vi "HOST_425.vi"() -> ()   [LabVIEW 2018]
uses:
  <vilib>/userdefined/High Color/nirio_resource_hc.ctl
  <instrlib>/niDCPower/nidcpower.llb/niDCPower Measurement Type.ctl
  <vilib>/FPGAPlugInAG/PXI-7953R/niLvFpga_Open_PXI-7953R.vi
  <vilib>/rvi/interface/common/dynamic/niFpgaDynamicAddResources.vi
  <vilib>/FPGAPlugInAG/Dynamic/niLvFpga_Reset_Dynamic.vi
  <vilib>/FPGAPlugInAG/Dynamic/niLvFpga_Run_Dynamic.vi
  <vilib>/Utility/error.llb/Error Cluster From Error Code.vi
  <vilib>/rvi/errors/niLvFpgaAdjustHostInterfaceError.vi
  <vilib>/FPGAPlugInAG/Dynamic/niLvFpga_Close_Dynamic.vi
  <vilib>/rvi/interface/nirviOpenFPGA/nirviOpenFPGA.xnode
  FPGA Bitfiles/IMX425LLJ_FPGATarget_Target0505_scNoFcOBk0w.lvbitx
  <vilib>/rvi/interface/nirviMethod/nirviMethod.xnode
  <vilib>/rvi/interface/nirviReadWriteControl/nirviReadWriteControl.xnode
  <vilib>/rvi/interface/nirviCloseFPGA/nirviCloseFPGA.xnode
  <vilib>/rvi/interface/Simulation/niFpgaSimulationCallBeginRW.vi
  <vilib>/FPGAPlugInAG/Dynamic/niLvFpga_ReadFifo_Dynamic.vi
  <vilib>/rvi/errors/niLvFpgaMergeErrorWithErrorCode.vi
  NiFpgaLv.dll
  <vilib>/FPGAPlugInAG/Dynamic/niLvFpga_StartFifo_Dynamic.vi
  <vilib>/FPGAPlugInAG/Dynamic/niLvFpga_WriteFifo_Dynamic.vi
panel:
  in  "Регистры":u32[](array[numeric])=[4194304, 4206720, 4205568, 4209664, 4197129, 4229936, 4213512, 4246304, 4205320, 4238224, 4221696, 4201291, 4233984, 4209536, 4212500, 4245304, 12582912, 12591104, 12623872, 12583936, 12616704, 12600320, 12633088, 12592128, 12624896, 12608512, 12641280, 12588032, 12620800, 12604416, 12637184, 12596224, 12628992, 12612608, 12645376, 12585984, 12618752, 12602368, 12635136, 12594176, 12626944, 12610560, 12643328, 12590080, 12622848, 12606464, 12639232, 12598272, 12631040, 12614656, 12647424, 12583424, 12616192, 12599808, 12632576, 12591616, 12624384, 12608000, 12640768, 12587520, 12620288, 12603904, 12636672, 12595712, 12628480, 12612096, 12644864, 12585472, 12618240, 12601856, 12634624, 12593664, 12626432, 12610048, 12642816, 12589568, 12622336, 12605952, 12638720, 12597760, 12630528, 12614144, 12646912, 2097188, 2105344, 2098186, 2130948, 2106378, 2139140, 2122949, 2100248, 2133016, 2116800, 2097716, 2130432, 2114048, 6291584, 6294656, 6335488, 6315008, 6306819, 6300352, 6332960, 6299136, 6331904, 6315520, 6348288, 6307328, 6340096, 6323712, 6291712, 6324480, 6308096, 6340864, 6299904, 6332672, 6316288, 14696448, 14682112, 14690304, 14723072, 14680892, 14713600, 14693320, 14725888, 14709688, 14742272, 1064960, 1097728, 1069064, 1101824, 1077288, 1110016, 1067248, 1099776, 1075296, 1107968, 1071152, 1103872, 1070080, 1102848, 1078288, 1111040, 1076264, 1108992, 1080362, 1113088, 1065520, 1098240, 1067520, 1100288, 1075728, 1108480, 1071624, 1104384, 1079848, 1112576, 1074784, 1107456, 13639680, 13632512, 13665344, 13648976, 13640959, 13673726, 13657088, 13636616, 13653000, 13644808, 13634645, 13667328, 13650950, 13683712, 13642752, 13675520, 13659136, 13691904, 13638656, 13671424, 13655040, 13687808, 13632192, 13664768, 15209792, 15242496]
  out "LED_char":dbl(graph)=-9.950040532110056e-06
  out "Память":i32
  out "Image":T1(plugin-control)
  in  "Хватит ждать!":bool
  out "Выкачали из памяти":bool
  out "SEU":u32
  in  "Upd_WR":bool
  out "FIFO_READ":u32
  in  "W(T)/R(F)":bool
  in  "Адрес":u8
  in  "Кол-во":u16=185
  out "НИ":bool
  out "READ":u8[](array[numeric])
  out "Прошили":bool
  in  "SPI":bool
  in  "Обнулить сбои":bool
  in  "Проверка сбоев":bool
  out "世男":bool
  in  "Период опроса, мс":u32=1
  in  "OVDD, V":dbl=1.8 caption="voltage level" format="%_6p"
  in  "OVDD_curlim":dbl=0.1 caption="current limit" format="%_6p"
  out "OVDD_char":dbl(graph)=1.5967060684808935e-06
  in  "3,3_LVDS, V":dbl=3.3 caption="voltage level" format="%_6p"
  in  "AVDD, V":dbl=3.3 caption="voltage level" format="%_6p"
  in  "DVDD, V":dbl=1.2 caption="voltage level" format="%_6p"
  in  "3,3_LVDS_curlim":dbl=0.2 caption="current limit" format="%_6p"
  in  "AVDD_curlim":dbl=1.0 caption="current limit" format="%_6p"
  in  "DVDD_curlim":dbl=1.0 caption="current limit" format="%_6p"
  in  "LED_curlim":dbl=0.1 caption="current limit" format="%_6p"
  in  "LED, V":dbl=-1.3 caption="voltage level" format="%_6p"
  out "3,3_LVDS_char":dbl(graph)=-0.007753012065680951
  out "AVDD_char":dbl(graph)=9.424895165128459e-05
  out "DVDD_char":dbl(graph)=-9.950040532110056e-06
  out "DVDD_cur":dbl caption="measurement" format="%_6g"
  out "LED_cur":dbl caption="measurement" format="%_6g"
  in  "SEL_Time, ms":u32=100
  in  "OVDD_selcur":dbl=0.01 caption="current limit" format="%_6p"
  in  "AVDD_selcur":dbl=0.6 caption="current limit" format="%_6p"
  in  "DVDD_selcur":dbl=0.9 caption="current limit" format="%_6p"
  out "AVDD_cur":dbl caption="measurement" format="%_6g"
  out "3,3_LVDS_cur":dbl caption="measurement" format="%_6g"
  out "OVDD_cur":dbl caption="measurement" format="%_6g"
  in  "MOVIE":bool
  in  "FRAME!":bool
  out "SEL":bool
  in  "SIM_SEL":bool
  out "OVDD":u16
  out "AVDD":u16
  out "DVDD":u16
  out "OVDD":bool
  out "AVDD":bool
  out "DVDD":bool
  in  "Стоп":bool
  in  "Питание":bool
  in  "LED":bool caption="output enabled"
  in  "0":refnum<k15>="PXI1Slot2" caption="1"
  in  "1":refnum<k15>="PXI1Slot3"
  in  "resource name 2":T2="PXI1Slot6"
  in  "SEU":path=path "C:/LabView_PRJ/GMAX0505/SEU"
  in  "SEL":path=path "C:/LabView_PRJ/GMAX0505/SEL"
  out "Номер образца":string="1"
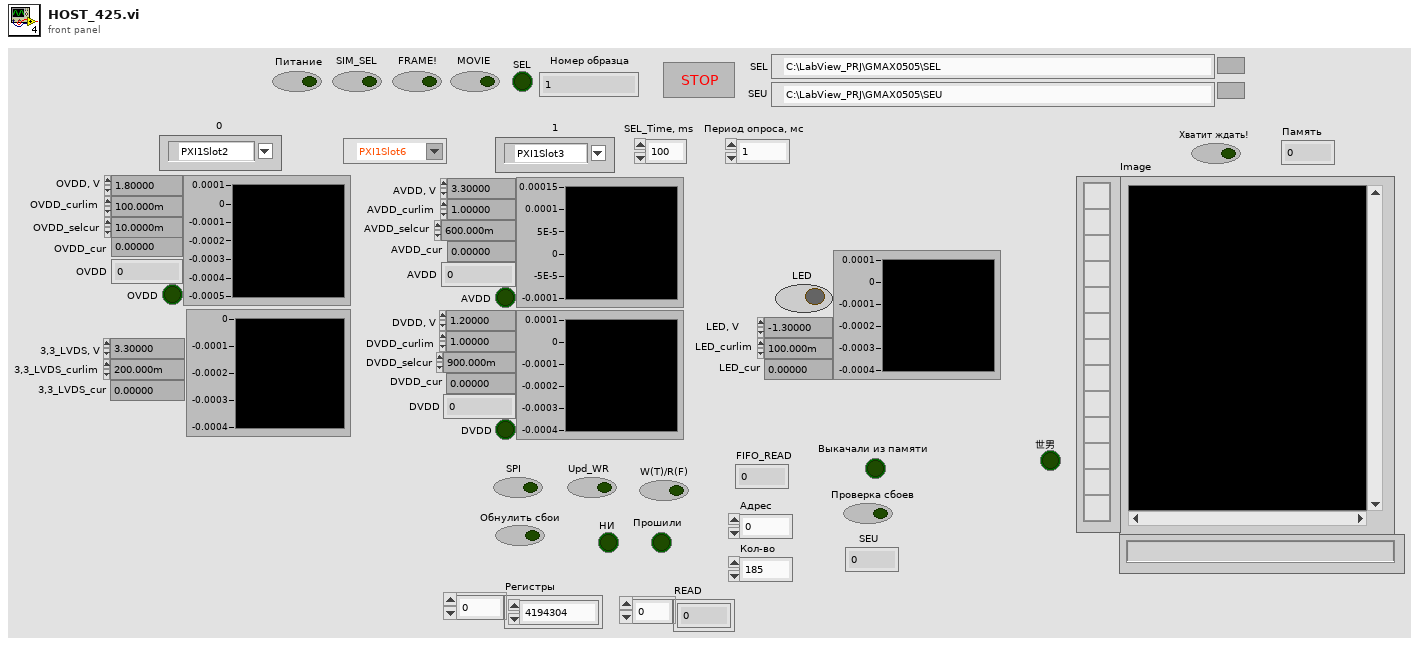
[diagram p1: front panel]
types:
  T1 = typedef "IMAQ Image.ctl" = refnum<image>
  T2 = typedef "nirio_resource_hc.ctl" = tag
  T3 = enum16{"open", "replace", "create", "open or create", "replace or create", "replace or create with confirmation"}
  T4 = typedef "Image Type" = u32
  T5 = typedef "niDCPower Measurement Type.ctl" = i32
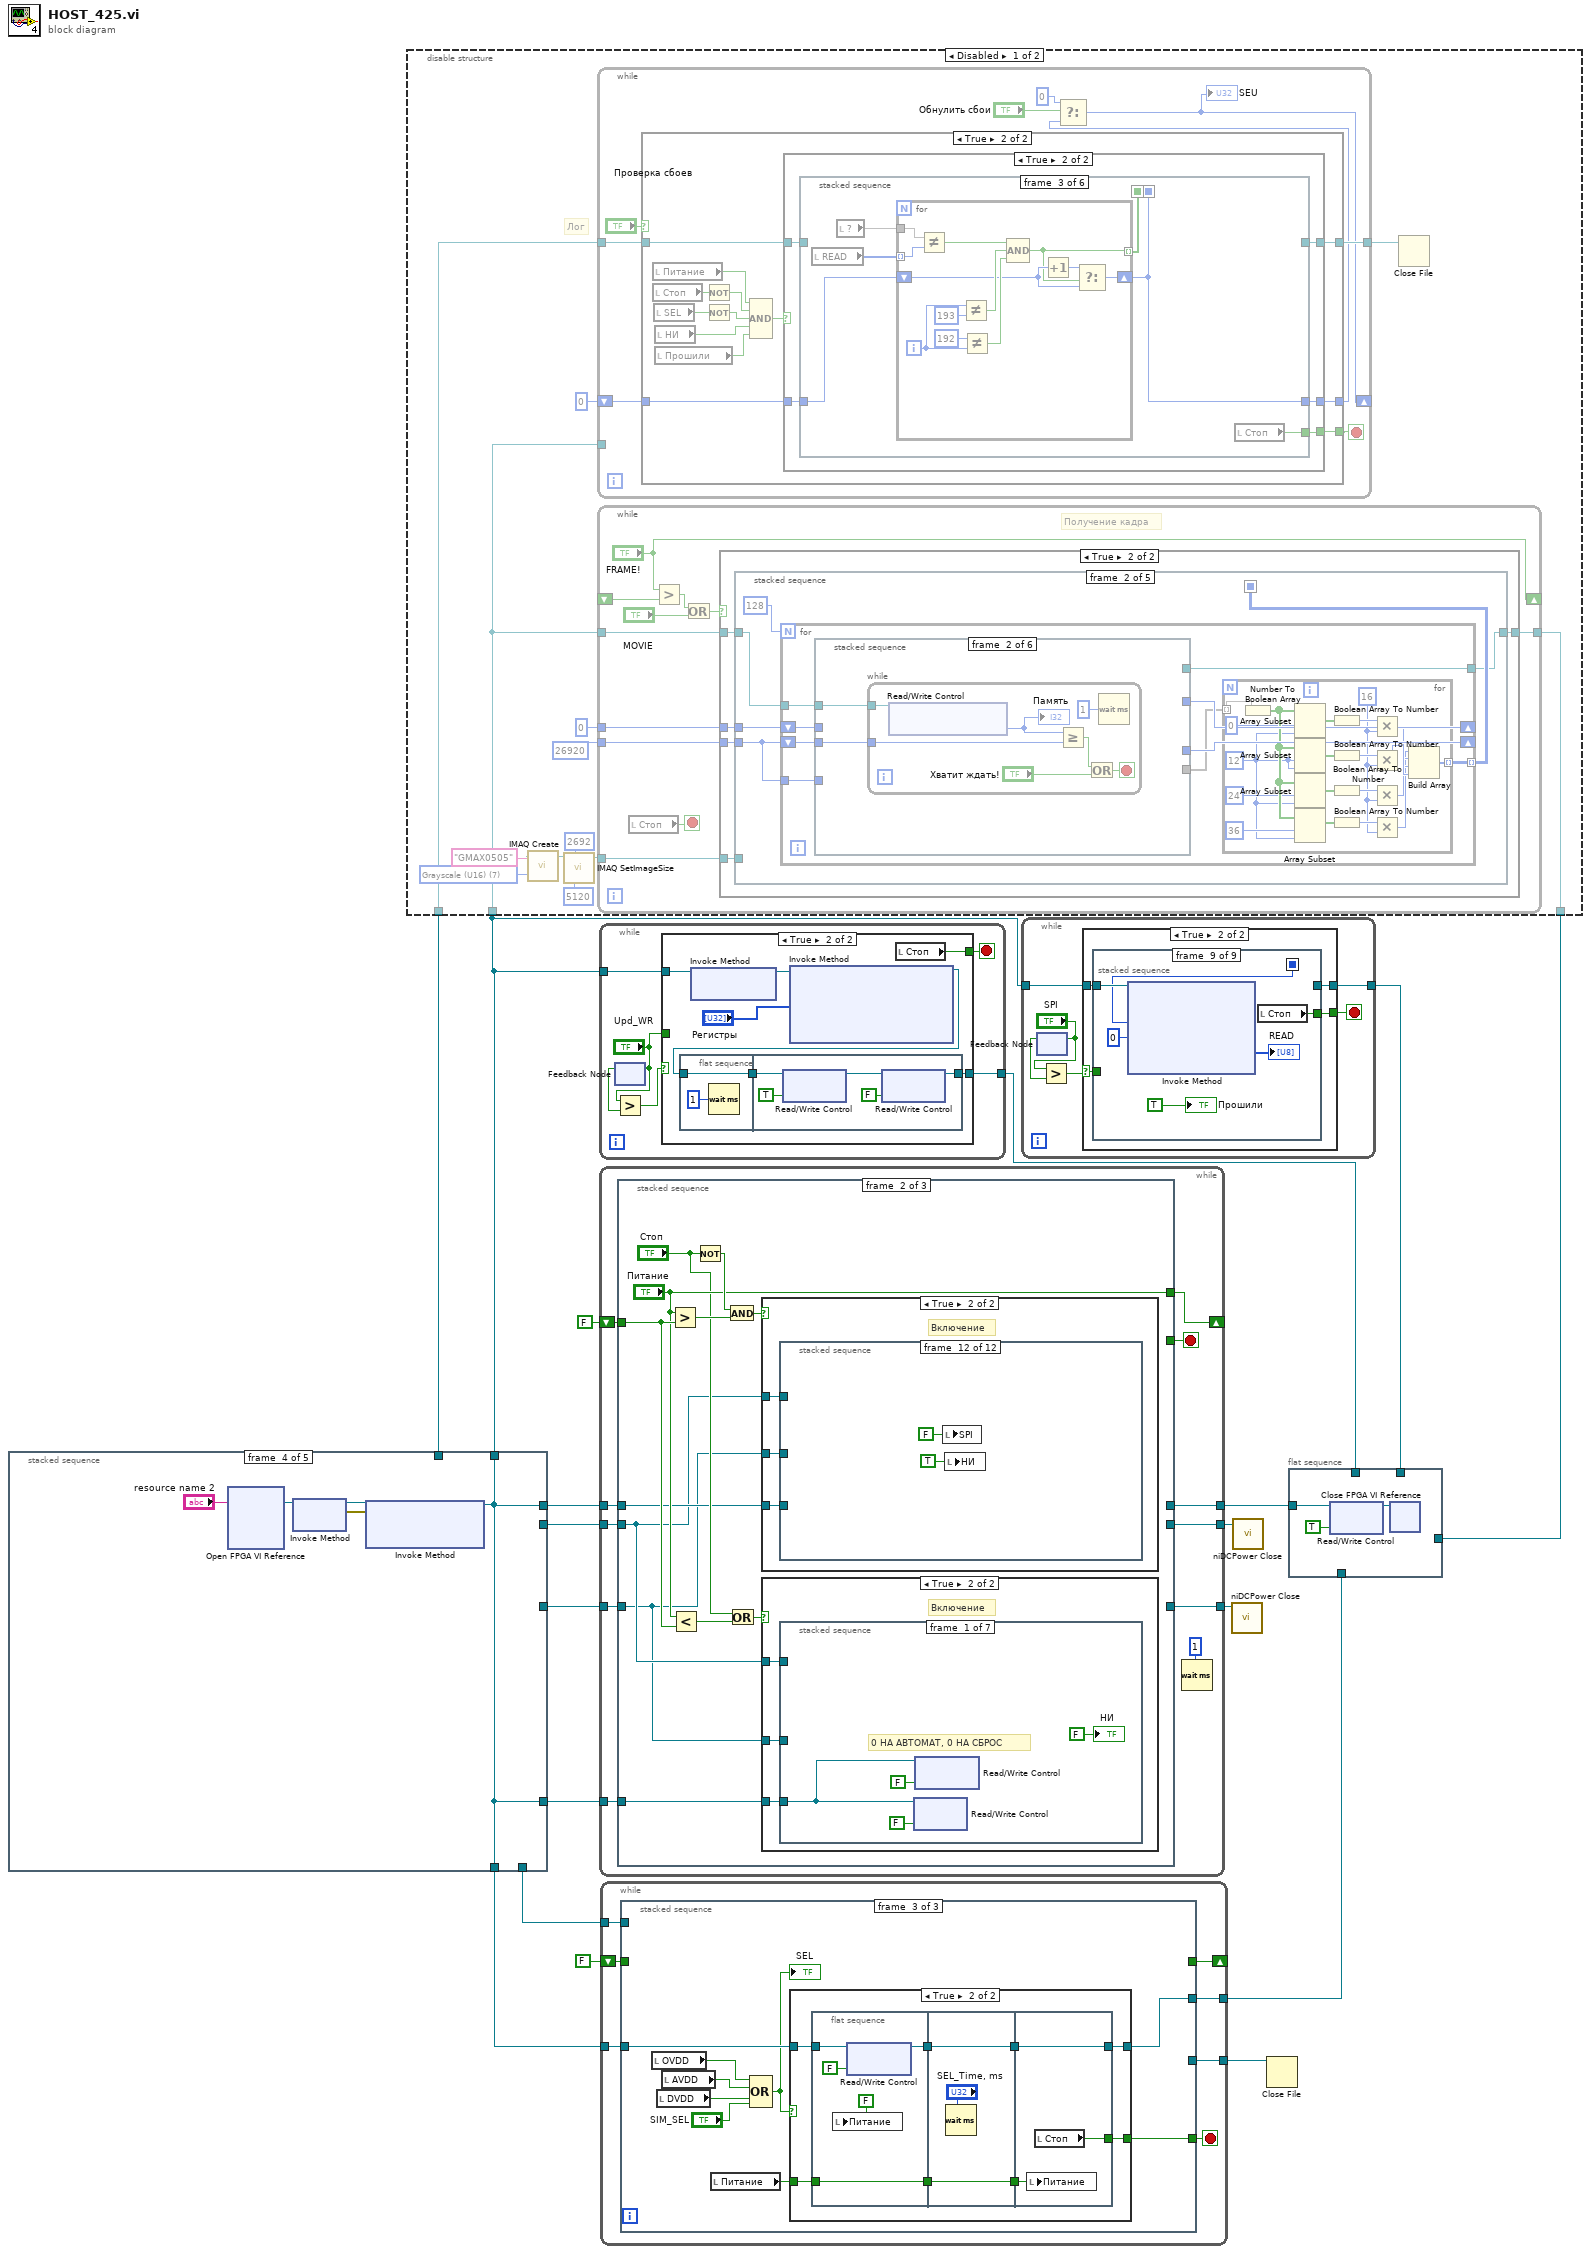
[diagram p0: block diagram]
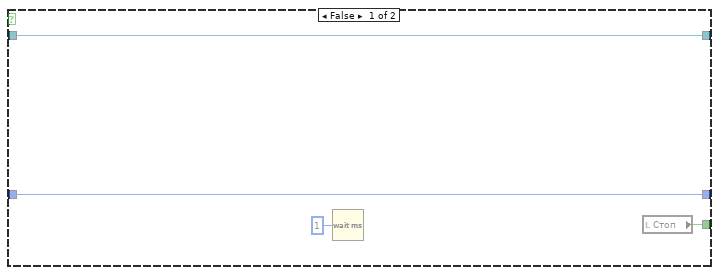
[diagram p2: hidden frame]
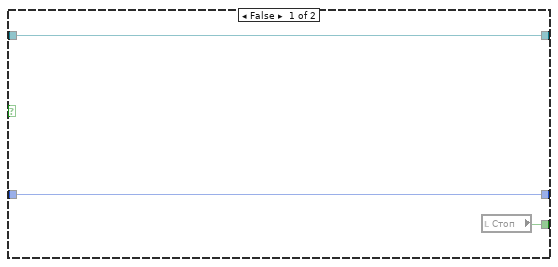
[diagram p3: hidden frame]
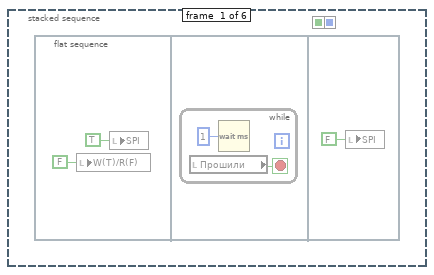
[diagram p4: hidden frame]
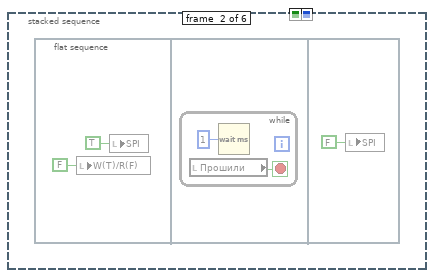
[diagram p5: hidden frame]
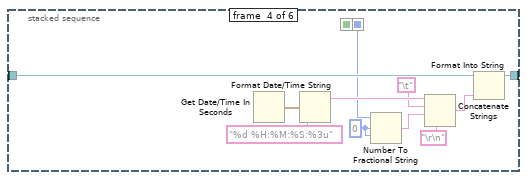
[diagram p6: hidden frame]
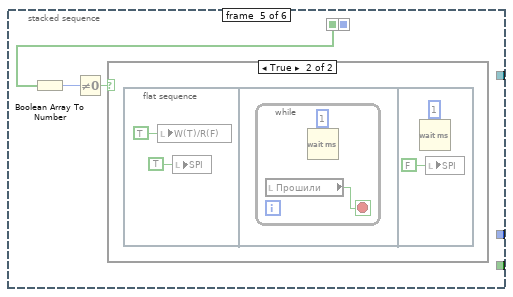
[diagram p7: hidden frame]
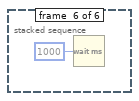
[diagram p9: hidden frame]
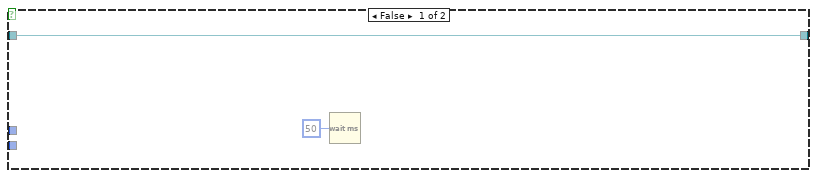
[diagram p10: hidden frame]
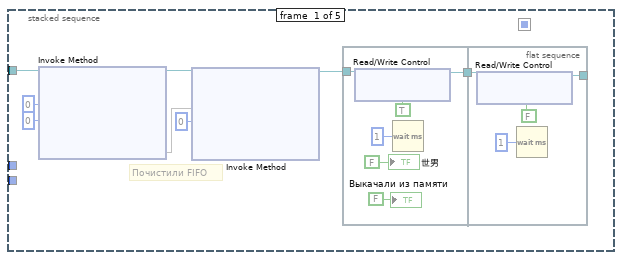
[diagram p11: hidden frame]
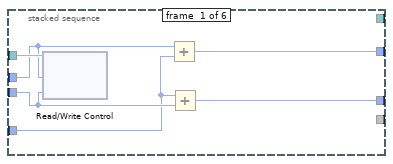
[diagram p12: hidden frame]
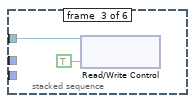
[diagram p13: hidden frame]
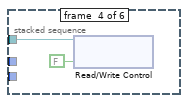
[diagram p14: hidden frame]
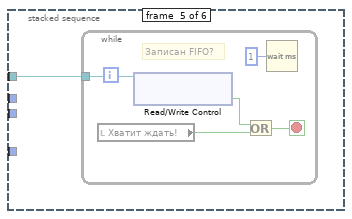
[diagram p15: hidden frame]
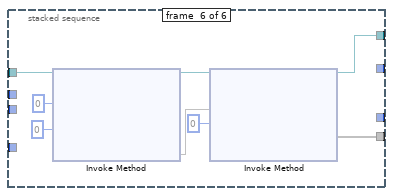
[diagram p16: hidden frame]
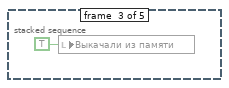
[diagram p17: hidden frame]
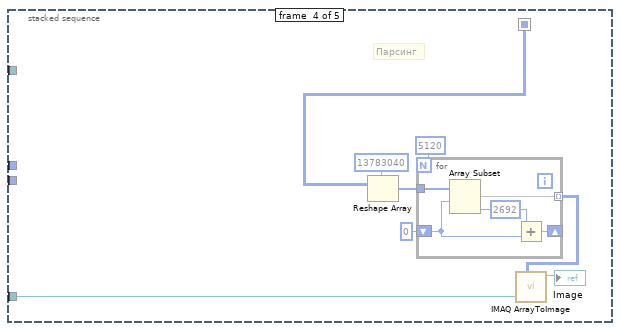
[diagram p18: hidden frame]
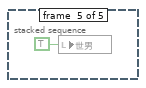
[diagram p19: hidden frame]
diagram:
  n1 = stacked-sequence {
    tunnel: [_ _ _ _ w90] -> w4
    tunnel: [_ _ _ _ w93] -> w3
    tunnel: [_ _ _ w85 _] -> w12
    tunnel: [_ _ _ w85 _] -> w15
    tunnel: [_ w26 _ _ _] -> w16
    tunnel: [_ _ _ w85 _] -> w10
    tunnel: [_ _ w54 _ _] -> w11
    tunnel: [_ _ _ w85 _] -> w8
    frame #0 {
      w19 = FALSE ("Стоп")
      w20 = FALSE ("Стоп")
      w21 = u16 0 ("ADC")
      # "Обнуление"
      n2 = call "Begin.vi"() -> ("Номер образца 2"=→"Номер образца":string)  [unwired: 11 in]
      n3 = local write "AVDD"(w19) -> ()
      n4 = local write "SIM_SEL"(w19) -> ()
      n5 = local write "SEL"(w19) -> ()
      n6 = local write "AVDD"(w21) -> ()
      n7 = local write "DVDD"(w21) -> ()
      n8 = local write "OVDD"(w21) -> ()
      n9 = local write "Стоп"(w20) -> ()
      n10 = local write "Питание"(w20) -> ()
      n11 = local write "FRAME!"(w20) -> ()
      n12 = local write "MOVIE"(w20) -> ()
      n13 = local write "LED"(w20) -> ()
      n14 = local write "Выкачали из памяти"(w20) -> ()
      n15 = local write "DVDD"(w20) -> ()
      n16 = local write "OVDD"(w20) -> ()
    }
    frame #1 {
      w25 = "\t"
      # "Лог по токам"
      n17 = local read "Номер образца"() -> (w46:string)
      n18 = Build Path(base path="SEL", name or relative path=w46) -> (appended path=w43:path)
      n19 = Get Date/Time In Seconds() -> (seconds since 1Jan1904=w40:timestamp)
      n20 = call <vilib>:"Check if File or Folder Exists.vi"("path"=w43) -> ("file or folder exists?"=w44:bool, "dup path"=w45:path)  [unwired: 8 in, 1 out]
      n21 = Format Date/Time String(time format string (%c)="%d %H.%M.%S", seconds (now)=w40) -> (date/time string=w38:string)  [unwired: 1 in]
      n22 = case shown="False" w44 {
        tunnel: w45 -> [w52 w53]
        tunnel: [w51 w53] -> w24
        frame False {
          n23 = Create Folder(path (use dialog)=w52) -> (created path=w51:path)  [unwired: 2 in, 2 out]
        }
        frame True {
        }
      }
      n24 = Concatenate Strings(w38, ".xls" ("string")) -> (w37:string)
      n25 = Build Path(base path=w24, name or relative path=w37) -> (appended path=w39:path)
      n26 = Open/Create/Replace File(file path (use dialog)=w39, operation (0:open)=T3."open or create", access (0:read/write)=enum16{"read/write", "read-only", "write-only"}."read/write") -> (refnum out=w41:refnum<file>)  [unwired: 3 in, 2 out]
      n27 = case shown="True" TRUE {
        tunnel: w41 -> [w47 w50]
        tunnel: [w47 w48] -> w36
        frame False {
        }
        frame True {
          n28 = Set File Position(refnum=w50, from (0:start)=enum16{"start", "end", "current"}."end") -> (refnum out=w48:refnum<file>)  [unwired: 2 in, 1 out]
        }
      }
      n29 = Format Into String(initial string=w36, "Time" ("input 1"), w25, "OVDD_cur", w25, "AVDD_cur", w25, "DVDD_cur", "\r\n") -> (resulting string=w26:refnum<file>)  [unwired: 2 in, 1 out]
    }
    frame #2 {
      w57 = "\t"
      # "Лог по сбоям"
      n30 = local read "Номер образца"() -> (w61:string)
      n31 = Build Path(base path="SEU", name or relative path=w61) -> (appended path=w75:path)
      n32 = Get Date/Time In Seconds() -> (seconds since 1Jan1904=w73:timestamp)
      n33 = call <vilib>:"Check if File or Folder Exists.vi"("path"=w75) -> ("file or folder exists?"=w76:bool, "dup path"=w77:path)  [unwired: 8 in, 1 out]
      n34 = Format Date/Time String(time format string (%c)="%d %H.%M.%S", seconds (now)=w73) -> (date/time string=w71:string)  [unwired: 1 in]
      n35 = case shown="False" w76 {
        tunnel: w77 -> [w83 w84]
        tunnel: [w82 w84] -> w62
        frame False {
          n36 = Create Folder(path (use dialog)=w83) -> (created path=w82:path)  [unwired: 2 in, 2 out]
        }
        frame True {
        }
      }
      n37 = Concatenate Strings(w71, ".xls" ("string")) -> (w70:string)
      n38 = Build Path(base path=w62, name or relative path=w70) -> (appended path=w72:path)
      n39 = Open/Create/Replace File(file path (use dialog)=w72, operation (0:open)=T3."open or create", access (0:read/write)=enum16{"read/write", "read-only", "write-only"}."read/write") -> (refnum out=w74:refnum<file>)  [unwired: 3 in, 2 out]
      n40 = case shown="True" TRUE {
        tunnel: w74 -> [w78 w81]
        tunnel: [w78 w79] -> w69
        frame False {
        }
        frame True {
          n41 = Set File Position(refnum=w81, from (0:start)=enum16{"start", "end", "current"}."end") -> (refnum out=w79:refnum<file>)  [unwired: 2 in, 1 out]
        }
      }
      n42 = Format Into String(initial string=w69, "Time" ("input 1"), w57, "Регистр №" ("input 3"), w57, "Содержание" ("input 4"), w57, "Кол-во сбоев" ("input 7"), "\r\n") -> (resulting string=w54:refnum<file>)  [unwired: 2 in, 1 out]
    }
    frame #3 {
      n43 = xnode "Open FPGA VI Reference"("resource name"="resource name 2") -> ("FPGA VI Reference Out"=w86:refnum<k20>)  [unwired: 1 in, 1 out]
      n44 = xnode "Invoke Method"("FPGA VI Reference In"=w86) -> ("FPGA VI Reference Out"=w89:refnum<k20>, "error out"=w88:errorcluster)  [unwired: 1 in]
      n45 = xnode "Invoke Method"("FPGA VI Reference In"=w89, "error in"=w88) -> ("FPGA VI Reference Out"=w85:refnum<k20>)  [unwired: 1 in, 1 out]
    }
    frame #4 {
      n46 = call <instrlib>:"niDCPower Initialize.vi"("resource name"="1") -> ("error out"=w96:errorcluster, "instrument handle out"=w94:refnum<k15>)  [unwired: 3 in, 6 out]
      n47 = call <instrlib>:"niDCPower Initialize.vi"("resource name"="0") -> ("error out"=w97:errorcluster, "instrument handle out"=w95:refnum<k15>)  [unwired: 3 in, 6 out]
      n48 = call <instrlib>:"niDCPower Configure Voltage Level.vi"("error in (no error)"=w96, "voltage level"=0.0, "channel name"="0,1,2", "instrument handle"=w94) -> ("instrument handle out"=w93:refnum<k15>)  [unwired: 6 in, 1 out]
      n49 = call <instrlib>:"niDCPower Configure Voltage Level.vi"("error in (no error)"=w97, "voltage level"=0.0, "channel name"="0,1", "instrument handle"=w95) -> ("instrument handle out"=w90:refnum<k15>)  [unwired: 6 in, 1 out]
    }
  }
  n50 = disable-structure shown="Disabled" {
    disable-tunnel: w12 -> [w108 _]
    disable-tunnel: w11 -> [w107 _]
    disable-tunnel: [w102 _] -> w5
    frame Disabled {
      w114 = T4 7 items=["Grayscale (U8)", "Grayscale (I16)", "Grayscale (SGL)", "Complex (CSG)", "RGB (U32)", "HSL (U32)", "RGB (U64)", "Grayscale (U16)"] ("Image Type")
      # "Лог"
      n51 = call "IMAQ Create"("Image Name"="GMAX0505", "Image Type"=w114) -> ("New Image"=w103:T1)  [unwired: 3 in, 1 out]
      n52 = call "IMAQ SetImageSize"("Y Resolution"=5120, "X Resolution"=2692, "Image"=w103) -> ("Image Out"=w106:T1)  [unwired: 2 in, 1 out]
      n53 = while {
        tunnel: w107 -> [w123]
        tunnel: [w122] -> w109
        shift-right: [w115] -> _
        shift-left: u32 0 -> [w119]
        tunnel: w108 -> [_]
        stop <- w120 stop-if-true
        n54 = case shown="True" "Проверка сбоев" {
          tunnel: [w125 w133] -> w120
          tunnel: w123 -> [w126 w134]
          tunnel: [w126 w130] -> w122
          tunnel: w119 -> [w124 w132]
          tunnel: [w124 w131] -> w117
          frame False {
            n55 = Wait (ms)(milliseconds to wait=u32 1) -> ()  [unwired: 1 out]
            n56 = local read "Стоп"() -> (w125:bool)
          }
          frame True {
            n57 = local read "Питание"() -> (w139:bool)
            n58 = local read "Стоп"() -> (w140:bool)
            n59 = local read "SEL"() -> (w129:bool)
            n60 = local read "НИ"() -> (w136:bool)
            n61 = local read "Прошили"() -> (w128:bool)
            n62 = Not(x=w140) -> (.not. x?=w138:bool)
            n63 = Not(x=w129) -> (.not. x?=w137:bool)
            n64 = Compound Arithmetic op=AND(w139, w138, w137, w136, w128) -> (w135:bool)
            n65 = case shown="True" w135 {
              tunnel: w134 -> [w141 w148]
              tunnel: [w143 w147] -> w133
              tunnel: w132 -> [w142 w146]
              tunnel: [w142 w145] -> w131
              tunnel: [w141 w144] -> w130
              frame False {
                n66 = local read "Стоп"() -> (w143:bool)
              }
              frame True {
                n67 = stacked-sequence {
                  seq-local: [_ _ w160 _ _ _] -> [_ _ _ w181 _ _]
                  seq-local: [_ _ w159 _ _ _] -> [_ _ _ _ w188 _]
                  tunnel: w148 -> [_ _ _ w186 _ _]
                  tunnel: [_ _ w164 _ _ _] -> w147
                  tunnel: w146 -> [_ _ w161 _ _ _]
                  tunnel: [_ _ w160 _ _ _] -> w145
                  tunnel: [_ _ _ w177 _ _] -> w144
                  frame #0 {
                    n68 = flat-sequence {
                      frame #0 {
                        n69 = local write "W(T)/R(F)"(FALSE ("W(T)/R(F)")) -> ()
                        n70 = local write "SPI"(TRUE ("SPI")) -> ()
                      }
                      frame #1 {
                        n71 = while {
                          stop <- w152 stop-if-true
                          n72 = local read "Прошили"() -> (w152:bool)
                          n73 = Wait (ms)(milliseconds to wait=u32 1) -> ()  [unwired: 1 out]
                        }
                      }
                      frame #2 {
                        n74 = local write "SPI"(FALSE ("SPI")) -> ()
                      }
                    }
                  }
                  frame #1 {
                    n75 = flat-sequence {
                      frame #0 {
                        n76 = local write "W(T)/R(F)"(FALSE ("W(T)/R(F)")) -> ()
                        n77 = local write "SPI"(TRUE ("SPI")) -> ()
                      }
                      frame #1 {
                        n78 = while {
                          stop <- w157 stop-if-true
                          n79 = local read "Прошили"() -> (w157:bool)
                          n80 = Wait (ms)(milliseconds to wait=u32 1) -> ()  [unwired: 1 out]
                        }
                      }
                      frame #2 {
                        n81 = local write "SPI"(FALSE ("SPI")) -> ()
                      }
                    }
                  }
                  frame #2 {
                    n82 = local read "READ"() -> (w163:u8[])
                    n83 = local read item#-1() -> (w162)
                    n84 = for {
                      tunnel: w163 -> [w169] mode=indexing
                      tunnel: w162 -> [w176]
                      shift-right: [w166] -> w160
                      shift-left: w161 -> [w167]
                      tunnel: [w165] -> w159 mode=indexing
                      i -> [w170]
                      n85 = Not Equal?(x=w176, y=w169) -> (x != y?=w173:bool)
                      n86 = Not Equal?(x=w170, y=193) -> (x != y?=w172:bool)
                      n87 = Not Equal?(x=192, y=w170) -> (x != y?=w171:bool)
                      n88 = Compound Arithmetic op=AND(w173, w172, w171) -> (w165:bool)
                      n89 = Increment(x=w167) -> (x+1=w168:u32)
                      n90 = Select(t=w168, s=w165, f=w167) -> (s? t:f=w166:u32)
                    }
                    n91 = local read "Стоп"() -> (w164:bool)
                  }
                  frame #3 {
                    w180 = i16 0 ("width (-)")
                    n92 = Get Date/Time In Seconds() -> (seconds since 1Jan1904=w185:timestamp)
                    n93 = Format Date/Time String(time format string (%c)="%d %H:%M:%S:%3u", seconds (now)=w185) -> (date/time string=w183:string)  [unwired: 1 in]
                    n94 = Number To Fractional String(number=w181, width (-)=w180, precision (6)=w180) -> (F-format string=w179:string)  [unwired: 1 in]
                    n95 = Concatenate Strings(w183, "\t", w179, "\r\n") -> (w187:string)
                    n96 = Format Into String(initial string=w186, w187) -> (resulting string=w177:refnum<file>)  [unwired: 2 in, 1 out]
                  }
                  frame #4 {
                    n97 = Boolean Array To Number(Boolean array=w188) -> (number=w190:u32)
                    n98 = Not Equal To 0?(x=w190) -> (x != 0?=w189:bool)
                    n99 = case shown="True" w189 {
                      frame False {
                      }
                      frame True {
                        n100 = flat-sequence {
                          frame #0 {
                            n101 = local write "W(T)/R(F)"(TRUE ("W(T)/R(F)")) -> ()
                            n102 = local write "SPI"(TRUE ("SPI")) -> ()
                          }
                          frame #1 {
                            n103 = while {
                              stop <- w194 stop-if-true
                              n104 = local read "Прошили"() -> (w194:bool)
                              n105 = Wait (ms)(milliseconds to wait=u32 1) -> ()  [unwired: 1 out]
                            }
                          }
                          frame #2 {
                            n106 = Wait (ms)(milliseconds to wait=u32 1) -> ()  [unwired: 1 out]
                            n107 = local write "SPI"(FALSE ("SPI")) -> ()
                          }
                        }
                      }
                    }
                  }
                  frame #5 {
                    n108 = Wait (ms)(milliseconds to wait=u32 1000) -> ()  [unwired: 1 out]
                  }
                }
              }
            }
          }
        }
        n109 = Select(t=u32 0, s="Обнулить сбои", f=w117) -> (s? t:f=w115:u32)
        "SEU" <- w115
      }
      n110 = while {
        tunnel: w108 -> [w205]
        shift-right: ["FRAME!"] -> _
        shift-left: _ -> [w208]
        tunnel: u32 0 -> [w204]
        tunnel: u32 26920 ("163840") -> [w203]
        tunnel: w106 -> [w199]
        tunnel: [w198] -> w102
        stop <- w202 stop-if-true
        # "Получение кадра"
        n111 = local read "Стоп"() -> (w202:bool)
        n112 = Greater?(x="FRAME!", y=w208) -> (0:w207:bool)
        n113 = Or(x=w207, y="MOVIE") -> (x .or. y?=w206:bool)
        n114 = case shown="True" w206 {
          tunnel: w205 -> [w209 w215]
          tunnel: w204 -> [_ w214]
          tunnel: w203 -> [_ w213]
          tunnel: w199 -> [_ w212]
          tunnel: [w209 w211] -> w198
          frame False {
            n115 = Wait (ms)(milliseconds to wait=u32 50) -> ()  [unwired: 1 out]
          }
          frame True {
            n116 = stacked-sequence {
              seq-local: [_ w235 _ _ _] -> [_ _ _ w303 _]
              tunnel: w215 -> [w219 w236 _ _ _]
              tunnel: w214 -> [_ w238 _ _ _]
              tunnel: w213 -> [_ w237 _ _ _]
              tunnel: w212 -> [_ _ _ w310 _]
              tunnel: [_ w234 _ _ _] -> w211
              frame #0 {
                # "Почистили FIFO"
                n117 = xnode "Invoke Method"("FPGA VI Reference In"=w219, "Number of Elements"=u32 0, "Timeout (ms)"=0) -> ("FPGA VI Reference Out"=w218:refnum<k20>, "Elements Remaining"=w220)  [unwired: 1 in, 2 out]
                n118 = xnode "Invoke Method"("FPGA VI Reference In"=w218, "Number of Elements"=w220, "Timeout (ms)"=0) -> ("FPGA VI Reference Out"=w217:refnum<k20>)  [unwired: 1 in, 3 out]
                n119 = flat-sequence {
                  tunnel: w217 -> [w229]
                  tunnel: [w225] -> w216
                  tunnel: [w231] -> _
                  tunnel: w216 -> [w230]
                  frame #0 {
                    n120 = xnode "Read/Write Control"("FPGA VI Reference In"=w229, "Кадр в память"=TRUE ("EXPOSURE")) -> ("FPGA VI Reference Out"=w225:refnum<k20>)  [unwired: 1 in, 1 out]
                    n121 = Wait (ms)(milliseconds to wait=u32 1) -> ()  [unwired: 1 out]
                    "世男" <- FALSE
                    "Выкачали из памяти" <- FALSE ("Выкачали из памяти")
                  }
                  frame #1 {
                    n122 = xnode "Read/Write Control"("FPGA VI Reference In"=w230, "Кадр в память"=FALSE) -> ("FPGA VI Reference Out"=w231:refnum<k20>)  [unwired: 1 in, 1 out]
                    n123 = Wait (ms)(milliseconds to wait=u32 1) -> ()  [unwired: 1 out]
                  }
                }
              }
              frame #1 {
                n124 = for {
                  N: 128 -> [_]
                  tunnel: w236 -> [w248]
                  shift-right: [w245] -> _
                  shift-left: w238 -> [w247]
                  shift-right: [w244] -> _
                  shift-left: w237 -> [w246]
                  tunnel: w237 -> [w243]
                  tunnel: [w241] -> w235 mode=indexing
                  tunnel: [w240] -> w234
                  n125 = stacked-sequence {
                    tunnel: w248 -> [w274 w275 w284 w286 w288 w294]
                    tunnel: w247 -> [w273 _ _ _ _ _]
                    tunnel: w246 -> [w272 w276 _ _ _ _]
                    tunnel: [w271 _ _ _ _ _] -> w245
                    tunnel: [w270 _ _ _ _ _] -> w244
                    tunnel: [_ _ _ _ _ w296] -> w242
                    tunnel: [_ _ _ _ _ w295] -> w240
                    tunnel: w243 -> [w269 _ _ _ _ _]
                    frame #0 {
                      n126 = xnode "Read/Write Control"("FPGA VI Reference In"=w274, "Нач_адр"=w273, "Кон_адр"=w272) -> ()  [unwired: 1 in, 2 out]
                      n127 = Add(x=w273, y=w269) -> (x+y=w271:u32)
                      n128 = Add(x=w269, y=w272) -> (x+y=w270:u32)
                    }
                    frame #1 {
                      n129 = while {
                        tunnel: w276 -> [w281]
                        tunnel: w275 -> [w279]
                        stop <- w280 stop-if-true
                        n130 = xnode "Read/Write Control"("FPGA VI Reference In"=w279) -> ("Записали адресов"=w277:u32)  [unwired: 1 in, 2 out]
                        "Память" <- w277
                        n131 = Greater Or Equal?(x=w277, y=w281) -> (x >= y?=w283:bool)
                        n132 = Or(x=w283, y="Хватит ждать!") -> (x .or. y?=w280:bool)
                        n133 = Wait (ms)(milliseconds to wait=u32 1) -> ()  [unwired: 1 out]
                      }
                    }
                    frame #2 {
                      n134 = xnode "Read/Write Control"("FPGA VI Reference In"=w284, "Кадр на ПК"=TRUE ("HOST")) -> ()  [unwired: 1 in, 2 out]
                    }
                    frame #3 {
                      n135 = xnode "Read/Write Control"("FPGA VI Reference In"=w286, "Кадр на ПК"=FALSE ("HOST")) -> ()  [unwired: 1 in, 2 out]
                    }
                    frame #4 {
                      n136 = while {
                        tunnel: w288 -> [w290]
                        stop <- w291 stop-if-true
                        # "Записан FIFO?"
                        n137 = local read "Хватит ждать!"() -> (w289:bool)
                        n138 = xnode "Read/Write Control"("FPGA VI Reference In"=w290) -> ("Записали FIFO"=w292:bool)  [unwired: 1 in, 2 out]
                        n139 = Or(x=w292, y=w289) -> (x .or. y?=w291:bool)
                        n140 = Wait (ms)(milliseconds to wait=u32 1) -> ()  [unwired: 1 out]
                      }
                    }
                    frame #5 {
                      n141 = xnode "Invoke Method"("FPGA VI Reference In"=w294, "Number of Elements"=u32 0, "Timeout (ms)"=0) -> ("FPGA VI Reference Out"=w300:refnum<k20>, "Elements Remaining"=w301)  [unwired: 1 in, 2 out]
                      n142 = xnode "Invoke Method"("FPGA VI Reference In"=w300, "Number of Elements"=w301, "Timeout (ms)"=0) -> ("FPGA VI Reference Out"=w295:refnum<k20>, "Data"=w296:void[])  [unwired: 1 in, 2 out]
                    }
                  }
                  n143 = for {
                    tunnel: w242 -> [w268] mode=indexing
                    tunnel: [w262] -> w241 mode=indexing
                    w253 = u16 16
                    w263 = 12 ("index")
                    n144 = Number To Boolean Array(number=w268) -> (Boolean array=w267:bool[])
                    n145 = Array Subset(array=w267, index=0, length=w263) -> (w261:bool[])
                    n146 = Array Subset(array=w267, index=w263, length=w263) -> (w260:bool[])
                    n147 = Array Subset(array=w267, index=24, length=w263) -> (w259:bool[])
                    n148 = Array Subset(array=w267, index=36, length=w263) -> (w258:bool[])
                    n149 = Boolean Array To Number(Boolean array=w261) -> (number=w257:u16)
                    n150 = Boolean Array To Number(Boolean array=w260) -> (number=w256:u16)
                    n151 = Boolean Array To Number(Boolean array=w259) -> (number=w255:u16)
                    n152 = Boolean Array To Number(Boolean array=w258) -> (number=w254:u16)
                    n153 = Multiply(x=w257, y=w253) -> (x*y=w252:u16)
                    n154 = Multiply(x=w256, y=w253) -> (x*y=w251:u16)
                    n155 = Multiply(x=w255, y=w253) -> (x*y=w250:u16)
                    n156 = Multiply(x=w254, y=w253) -> (x*y=w249:u16)
                    n157 = Build Array(w249, w250, w251, w252) -> (w262:u16[])
                  }
                }
              }
              frame #2 {
                n158 = local write "Выкачали из памяти"(TRUE ("Выкачали из памяти")) -> ()
              }
              frame #3 {
                # "Парсинг"
                n159 = Reshape Array(w303, 13783040 ("dimension size")) -> (w308:u16[])
                n160 = for {
                  N: 5120 ("6032") -> [_]
                  shift-right: [w315] -> _
                  shift-left: 0 ("index") -> [w314]
                  tunnel: [w313] -> w307 mode=indexing
                  tunnel: w308 -> [w311]
                  w312 = 2692 ("3964")
                  n161 = Array Subset(array=w311, index=w314, length=w312) -> (w313:u16[])
                  n162 = Add(x=w312, y=w314) -> (x+y=w315:i32)
                }
                n163 = call "IMAQ ArrayToImage"("Image Pixels (U16)"=w307, "Image"=w310) -> ("Image Out"=→"Image":T1)  [unwired: 8 in, 1 out]
              }
              frame #4 {
                n164 = local write "世男"(TRUE ("世男")) -> ()
              }
            }
          }
        }
      }
      n165 = Close File(refnum=w109) -> ()  [unwired: 1 in, 2 out]
    }
    frame Enabled {
    }
  }
  n166 = while {
    tunnel: w12 -> [w319]
    tunnel: [w317] -> w6
    stop <- w321 stop-if-true
    n167 = feedback-in #1("Upd_WR") -> ()
    n168 = feedback #1() -> (w322:bool)  [unwired: 1 in]
    n169 = Greater?(x="Upd_WR", y=w322) -> (0:w320:bool)
    n170 = case shown="True" w320 {
      tunnel: [w324 w332] -> w321
      tunnel: w319 -> [w323 w329]
      tunnel: "Upd_WR" -> [_ _]
      tunnel: [w323 w327] -> w317
      frame False {
        n171 = Wait (ms)(milliseconds to wait=u32 50) -> ()  [unwired: 1 out]
        n172 = local read "Стоп"() -> (w324:bool)
      }
      frame True {
        n173 = flat-sequence {
          tunnel: w331 -> [w334]
          tunnel: [w334] -> w328
          tunnel: w328 -> [w339]
          tunnel: [w335] -> w327
          frame #0 {
            n174 = Wait (ms)(milliseconds to wait=u32 1) -> ()  [unwired: 1 out]
          }
          frame #1 {
            n175 = xnode "Read/Write Control"("FPGA VI Reference In"=w339, "Upd_WR"=TRUE) -> ("FPGA VI Reference Out"=w338:refnum<k20>)  [unwired: 1 in, 1 out]
            n176 = xnode "Read/Write Control"("FPGA VI Reference In"=w338, "Upd_WR"=FALSE) -> ("FPGA VI Reference Out"=w335:refnum<k20>)  [unwired: 1 in, 1 out]
          }
        }
        n177 = xnode "Invoke Method"("FPGA VI Reference In"=w329) -> ("FPGA VI Reference Out"=w330:refnum<k20>)  [unwired: 1 in, 1 out]
        n178 = xnode "Invoke Method"("FPGA VI Reference In"=w330, "Data"="Регистры") -> ("FPGA VI Reference Out"=w331:refnum<k20>)  [unwired: 2 in, 2 out]
        n179 = local read "Стоп"() -> (w332:bool)
      }
    }
  }
  n180 = while {
    shift-right: [w349] -> _
    shift-left: FALSE -> [w350]
    tunnel: w10 -> [w346]
    tunnel: [w345] -> w9
    tunnel: w8 -> [w344]
    tunnel: w4 -> [w343]
    tunnel: w3 -> [w342]
    tunnel: [w341] -> w2
    tunnel: [w340] -> w1
    stop <- w348 stop-if-true
    n181 = stacked-sequence {
      tunnel: w350 -> [_ w408 _]
      tunnel: [_ "Питание" _] -> w349
      tunnel: [_ _ w460] -> w348
      tunnel: w346 -> [_ w400 w459]
      tunnel: [_ _ w459] -> w345
      tunnel: w344 -> [_ w399 _]
      tunnel: w343 -> [w353 w398 w458]
      tunnel: w342 -> [w352 w397 w457]
      tunnel: [_ _ w458] -> w341
      tunnel: [_ _ w457] -> w340
      frame #0 {
        w354 = T5 0 items=["Current", "Voltage"] ("measurement type")
        n182 = call <instrlib>:"niDCPower Configure Current Limit.vi"("current limit"="OVDD_curlim", "channel name"="0", "instrument handle"=w353) -> ("instrument handle out"=w365:refnum<k15>)  [unwired: 7 in, 1 out]
        n183 = call <instrlib>:"niDCPower Configure Current Limit.vi"("current limit"="3,3_LVDS_curlim", "channel name"="1", "instrument handle"=w353) -> ("instrument handle out"=w384:refnum<k15>)  [unwired: 7 in, 1 out]
        n184 = call <instrlib>:"niDCPower Configure Current Limit.vi"("current limit"="AVDD_curlim", "channel name"="0", "instrument handle"=w352) -> ("instrument handle out"=w385:refnum<k15>)  [unwired: 7 in, 1 out]
        n185 = call <instrlib>:"niDCPower Configure Current Limit.vi"("current limit"="DVDD_curlim", "channel name"="1", "instrument handle"=w352) -> ("instrument handle out"=w386:refnum<k15>)  [unwired: 7 in, 1 out]
        n186 = call <instrlib>:"niDCPower Configure Current Limit.vi"("current limit"="LED_curlim", "channel name"="2", "instrument handle"=w352) -> ("instrument handle out"=w387:refnum<k15>)  [unwired: 7 in, 1 out]
        n187 = call <instrlib>:"niDCPower Configure Voltage Level.vi"("voltage level"="OVDD, V", "channel name"="0", "instrument handle"=w365) -> ("instrument handle out"=w368:refnum<k15>)  [unwired: 7 in, 1 out]
        n188 = call <instrlib>:"niDCPower Configure Voltage Level.vi"("voltage level"="3,3_LVDS, V", "channel name"="1", "instrument handle"=w384) -> ("instrument handle out"=w372:refnum<k15>)  [unwired: 7 in, 1 out]
        n189 = call <instrlib>:"niDCPower Configure Voltage Level.vi"("voltage level"="AVDD, V", "channel name"="0", "instrument handle"=w385) -> ("instrument handle out"=w371:refnum<k15>)  [unwired: 7 in, 1 out]
        n190 = call <instrlib>:"niDCPower Configure Voltage Level.vi"("voltage level"="DVDD, V", "channel name"="1", "instrument handle"=w386) -> ("instrument handle out"=w370:refnum<k15>)  [unwired: 7 in, 1 out]
        n191 = call <instrlib>:"niDCPower Configure Voltage Level.vi"("voltage level"="LED, V", "channel name"="2", "instrument handle"=w387) -> ("instrument handle out"=w356:refnum<k15>)  [unwired: 7 in, 1 out]
        n192 = call <instrlib>:"niDCPower Measure.vi"("measurement type"=w354, "channel name"="0", "instrument handle"=w368) -> ("measurement"=→"OVDD_char" →"OVDD_cur":dbl)  [unwired: 6 in, 2 out]
        n193 = call <instrlib>:"niDCPower Measure.vi"("measurement type"=w354, "channel name"="1", "instrument handle"=w372) -> ("measurement"=→"3,3_LVDS_char" →"3,3_LVDS_cur":dbl)  [unwired: 6 in, 2 out]
        n194 = call <instrlib>:"niDCPower Measure.vi"("measurement type"=w354, "channel name"="0", "instrument handle"=w371) -> ("measurement"=→"AVDD_char" →"AVDD_cur":dbl)  [unwired: 6 in, 2 out]
        n195 = call <instrlib>:"niDCPower Measure.vi"("measurement type"=w354, "channel name"="1", "instrument handle"=w370) -> ("measurement"=→"DVDD_char" →"DVDD_cur":dbl)  [unwired: 6 in, 2 out]
        n196 = call <instrlib>:"niDCPower Configure Output Enabled.vi"("output enabled"="LED", "channel name"="2", "instrument handle"=w356) -> ("instrument handle out"=w355:refnum<k15>)  [unwired: 7 in, 1 out]
        n197 = call <instrlib>:"niDCPower Measure.vi"("measurement type"=w354, "channel name"="2", "instrument handle"=w355) -> ("measurement"=→"LED_cur" →"LED_char":dbl)  [unwired: 6 in, 2 out]
      }
      frame #1 {
        n198 = Greater?(x="Питание", y=w408) -> (0:w406:bool)
        n199 = Less?(x="Питание", y=w408) -> (x < y?=w404:bool)
        n200 = Not(x="Стоп") -> (.not. x?=w405:bool)
        n201 = And(x=w405, y=w406) -> (x .and. y?=w407:bool)
        n202 = Or(x="Стоп", y=w404) -> (x .or. y?=w402:bool)
        n203 = case shown="True" w407 {
          tunnel: w400 -> [_ w430]
          tunnel: w398 -> [_ w429]
          tunnel: w397 -> [_ w428]
          frame False {
          }
          frame True {
            # "Включение"
            n204 = stacked-sequence {
              tunnel: w430 -> [_ _ _ _ _ _ w447 _ w450 _ _ _]
              tunnel: w429 -> [_ _ w435 _ w439 _ _ _ _ _ _ _]
              tunnel: w428 -> [w431 _ _ _ w442 _ _ _ _ _ _ _]
              frame #0 {
                # "DVDD"
                n205 = call <instrlib>:"niDCPower Configure Output Enabled.vi"("output enabled"=TRUE, "channel name"="1", "instrument handle"=w431) -> ()  [unwired: 7 in, 2 out]
              }
              frame #1 {
                n206 = Wait (ms)(milliseconds to wait=u32 50) -> ()  [unwired: 1 out]
              }
              frame #2 {
                # "OVDD"
                n207 = call <instrlib>:"niDCPower Configure Output Enabled.vi"("output enabled"=TRUE, "channel name"="0", "instrument handle"=w435) -> ()  [unwired: 7 in, 2 out]
              }
              frame #3 {
                n208 = Wait (ms)(milliseconds to wait=u32 50) -> ()  [unwired: 1 out]
              }
              frame #4 {
                # "LVDS"
                # "AVDD"
                n209 = call <instrlib>:"niDCPower Configure Output Enabled.vi"("output enabled"=TRUE, "channel name"="1", "instrument handle"=w439) -> ()  [unwired: 7 in, 2 out]
                n210 = call <instrlib>:"niDCPower Configure Output Enabled.vi"("output enabled"=TRUE, "channel name"="0", "instrument handle"=w442) -> ()  [unwired: 7 in, 2 out]
              }
              frame #5 {
                n211 = Wait (ms)(milliseconds to wait=u32 50) -> ()  [unwired: 1 out]
              }
              frame #6 {
                # "XCLR В ЕДНИЦУ"
                n212 = xnode "Read/Write Control"("FPGA VI Reference In"=w447, "XCLR"=TRUE ("Автомат")) -> ()  [unwired: 1 in, 2 out]
              }
              frame #7 {
                n213 = Wait (ms)(milliseconds to wait=u32 1) -> ()  [unwired: 1 out]
              }
              frame #8 {
                # "ВКЛЮЧАЕМ ТАКТОВУЮ"
                n214 = xnode "Read/Write Control"("FPGA VI Reference In"=w450, "Автомат"=TRUE) -> ()  [unwired: 1 in, 2 out]
              }
              frame #9 {
                n215 = Wait (ms)(milliseconds to wait=u32 1) -> ()  [unwired: 1 out]
              }
              frame #10 {
                # "Прошиваем регистры"
                n216 = local write "SPI"(TRUE ("SPI")) -> ()
                n217 = local write "W(T)/R(F)"(TRUE ("SPI")) -> ()
                n218 = Wait (ms)(milliseconds to wait=u32 10) -> ()  [unwired: 1 out]
              }
              frame #11 {
                n219 = local write "SPI"(FALSE ("SPI")) -> ()
                n220 = local write "НИ"(TRUE ("НИ")) -> ()
              }
            }
          }
        }
        n221 = case shown="True" w402 {
          tunnel: w399 -> [_ w411]
          tunnel: w398 -> [_ w410]
          tunnel: w397 -> [_ w409]
          frame False {
          }
          frame True {
            # "Включение"
            n222 = stacked-sequence {
              tunnel: w411 -> [w414 _ _ _ _ _ _]
              tunnel: w410 -> [_ _ _ _ w421 _ _]
              tunnel: w409 -> [_ _ w417 _ _ _ w425]
              frame #0 {
                # "0 НА АВТОМАТ, 0 НА СБРОС"
                n223 = xnode "Read/Write Control"("FPGA VI Reference In"=w414, "XCLR"=FALSE) -> ()  [unwired: 1 in, 2 out]
                n224 = xnode "Read/Write Control"("FPGA VI Reference In"=w414, "Автомат"=FALSE) -> ()  [unwired: 1 in, 2 out]
                "НИ" <- FALSE ("НИ")
              }
              frame #1 {
                n225 = Wait (ms)(milliseconds to wait=u32 1) -> ()  [unwired: 1 out]
              }
              frame #2 {
                # "AVDD"
                n226 = call <instrlib>:"niDCPower Configure Output Enabled.vi"("output enabled"=FALSE, "channel name"="0", "instrument handle"=w417) -> ()  [unwired: 7 in, 2 out]
              }
              frame #3 {
                n227 = Wait (ms)(milliseconds to wait=u32 50) -> ()  [unwired: 1 out]
              }
              frame #4 {
                # "OVDD"
                n228 = call <instrlib>:"niDCPower Configure Output Enabled.vi"("output enabled"=FALSE, "channel name"="0", "instrument handle"=w421) -> ()  [unwired: 7 in, 2 out]
              }
              frame #5 {
                n229 = Wait (ms)(milliseconds to wait=u32 50) -> ()  [unwired: 1 out]
              }
              frame #6 {
                # "VDD13"
                n230 = call <instrlib>:"niDCPower Configure Output Enabled.vi"("output enabled"=FALSE, "channel name"="1", "instrument handle"=w425) -> ()  [unwired: 7 in, 2 out]
              }
            }
          }
        }
      }
      frame #2 {
        n231 = local read "Стоп"() -> (w460:bool)
      }
    }
    n232 = Wait (ms)(milliseconds to wait=u32 1) -> ()  [unwired: 1 out]
  }
  n233 = while {
    tunnel: w15 -> [w463]
    shift-right: [w466] -> _
    shift-left: FALSE ("Питание") -> [w467]
    tunnel: w16 -> [w465]
    tunnel: [w462] -> w17
    tunnel: [w461] -> w13
    stop <- w464 stop-if-true
    n234 = stacked-sequence {
      tunnel: w467 -> [w471 _ _]
      tunnel: [w470 _ _] -> w466
      tunnel: w465 -> [_ w515 _]
      tunnel: [_ _ w527] -> w464
      tunnel: w463 -> [_ _ w526]
      tunnel: [_ w508 _] -> w462
      tunnel: [_ _ w524] -> w461
      frame #0 {
        n235 = flat-sequence {
          tunnel: w469 -> [w472]
          frame #0 {
            n236 = case shown="True" w472 {
              frame False {
              }
              frame True {
                n237 = Wait (ms)(milliseconds to wait=u32 500) -> ()  [unwired: 1 out]
              }
            }
          }
          frame #1 {
            n238 = local read "AVDD_cur"() -> (w478:dbl)
            n239 = local read "DVDD_cur"() -> (w479:dbl)
            n240 = local read "OVDD_cur"() -> (w477:dbl)
            n241 = Greater Or Equal?(x=w478, y="AVDD_selcur") -> (x >= y?=w475:bool)
            "AVDD" <- w475
            n242 = Greater Or Equal?(x=w477, y="OVDD_selcur") -> (x >= y?=w476:bool)
            "OVDD" <- w476
            n243 = Greater Or Equal?(x=w479, y="DVDD_selcur") -> (x >= y?=w474:bool)
            "DVDD" <- w474
            n244 = case shown="True" w476 {
              frame False {
              }
              frame True {
                n245 = local read "OVDD"() -> (w487:u16)
                n246 = Increment(x=w487) -> (x+1=→"OVDD":u16)
              }
            }
            n247 = case shown="True" w474 {
              frame False {
              }
              frame True {
                n248 = local read "DVDD"() -> (w483:u16)
                n249 = Increment(x=w483) -> (x+1=→"DVDD":u16)
              }
            }
            n250 = case shown="True" w475 {
              frame False {
              }
              frame True {
                n251 = local read "AVDD"() -> (w485:u16)
                n252 = Increment(x=w485) -> (x+1=→"AVDD":u16)
              }
            }
          }
        }
        n253 = local read "Питание"() -> (w470:bool)
        n254 = Greater?(x=w470, y=w471) -> (0:w469:bool)
        n255 = Wait (ms)(milliseconds to wait="Период опроса, мс") -> ()  [unwired: 1 out]
      }
      frame #1 {
        w501 = "\t"
        w503 = i16 0 ("width (-)")
        w507 = i16 3 ("width (-)")
        n256 = local read "OVDD_cur"() -> (w514:dbl)
        n257 = local read "AVDD, V"() -> (w513:dbl)
        n258 = local read "DVDD_cur"() -> (w502:dbl)
        n259 = local read "OVDD"() -> (w506:u16)
        n260 = local read "AVDD"() -> (w505:u16)
        n261 = local read "DVDD"() -> (w504:u16)
        n262 = Get Date/Time In Seconds() -> (seconds since 1Jan1904=w518:timestamp)
        n263 = Format Date/Time String(time format string (%c)="%d %H:%M:%S:%3u", seconds (now)=w518) -> (date/time string=w512:string)  [unwired: 1 in]
        n264 = Number To Fractional String(number=w514, width (-)=w507, precision (6)=w507) -> (F-format string=w511:string)  [unwired: 1 in]
        n265 = Number To Fractional String(number=w513, width (-)=w507, precision (6)=w507) -> (F-format string=w510:string)  [unwired: 1 in]
        n266 = Number To Fractional String(number=w502, width (-)=w507, precision (6)=w507) -> (F-format string=w509:string)  [unwired: 1 in]
        n267 = Number To Fractional String(number=w506, width (-)=w503, precision (6)=w503) -> (F-format string=w500:string)  [unwired: 1 in]
        n268 = Number To Fractional String(number=w505, width (-)=w503, precision (6)=w503) -> (F-format string=w499:string)  [unwired: 1 in]
        n269 = Number To Fractional String(number=w504, width (-)=w503, precision (6)=w503) -> (F-format string=w498:string)  [unwired: 1 in]
        n270 = local read "OVDD"() -> (w496:bool)
        n271 = local read "AVDD"() -> (w495:bool)
        n272 = local read "DVDD"() -> (w494:bool)
        n273 = local read "SIM_SEL"() -> (w493:bool)
        n274 = Compound Arithmetic op=OR(w496, w495, w494, w493) -> (w497:bool)
        n275 = Select(t="!!!", s=w497, f="") -> (s? t:f=w490:string)
        n276 = Concatenate Strings(w512, w501, w511, w501, w510, w501, w509, w501, w500, w501, w499, w501, w498, w501, w490, "\r\n") -> (w516:string)
        n277 = Format Into String(initial string=w515, w516) -> (resulting string=w508:refnum<file>)  [unwired: 2 in, 1 out]
      }
      frame #2 {
        n278 = local read "OVDD"() -> (w522:bool)
        n279 = local read "DVDD"() -> (w520:bool)
        n280 = local read "AVDD"() -> (w521:bool)
        n281 = local read "Питание"() -> (w525:bool)
        n282 = Compound Arithmetic op=OR(w522, w521, w520, "SIM_SEL") -> (w523:bool)
        "SEL" <- w523
        n283 = case shown="True" w523 {
          tunnel: [w529 w537] -> w527
          tunnel: w526 -> [w528 w536]
          tunnel: w525 -> [_ w533]
          tunnel: [w528 w532] -> w524
          frame False {
            n284 = local read "Стоп"() -> (w529:bool)
          }
          frame True {
            n285 = flat-sequence {
              tunnel: w536 -> [w541]
              tunnel: [w539] -> w534
              tunnel: w533 -> [w539]
              tunnel: [w538] -> w530
              tunnel: [w544] -> w535
              tunnel: w534 -> [w544]
              tunnel: [w543] -> w531
              tunnel: w530 -> [w543]
              tunnel: [w548] -> w537
              tunnel: w535 -> [w547]
              tunnel: [w546] -> w532
              tunnel: w531 -> [w546]
              frame #0 {
                n286 = local write "Питание"(FALSE ("Питание")) -> ()
                n287 = xnode "Read/Write Control"("FPGA VI Reference In"=w541, "Автомат"=FALSE ("Линейки")) -> ("FPGA VI Reference Out"=w538:refnum<k20>)  [unwired: 1 in, 1 out]
              }
              frame #1 {
                n288 = Wait (ms)(milliseconds to wait="SEL_Time, ms") -> ()  [unwired: 1 out]
              }
              frame #2 {
                n289 = local write "Питание"(w547) -> ()
                n290 = local read "Стоп"() -> (w548:bool)
              }
            }
          }
        }
      }
    }
  }
  n291 = while {
    tunnel: w12 -> [w552]
    tunnel: [w550] -> w7
    stop <- w551 stop-if-true
    n292 = feedback #2() -> (w554:bool)  [unwired: 1 in]
    n293 = feedback-in #2("SPI") -> ()
    n294 = Greater?(x="SPI", y=w554) -> (0:w553:bool)
    n295 = case shown="True" w553 {
      selector: w553 -> [_ w560]
      tunnel: w552 -> [w555 w561]
      tunnel: [w557 w559] -> w551
      tunnel: [w555 w558] -> w550
      frame False {
        n296 = Wait (ms)(milliseconds to wait=u32 1) -> ()  [unwired: 1 out]
        n297 = local read "Стоп"() -> (w557:bool)
      }
      frame True {
        n298 = stacked-sequence {
          seq-local: [_ _ _ _ _ _ _ w578 _] -> [_ _ _ _ _ _ _ _ w585]
          tunnel: w561 -> [w567 _ w570 _ w574 _ w577 w581 w586]
          tunnel: w560 -> [_ _ _ _ _ _ _ _ _]
          tunnel: [_ _ _ _ _ _ _ _ w587] -> w559
          tunnel: [w563 _ _ _ _ _ _ _ _] -> w558
          frame #0 {
            n299 = local write "Прошили"(FALSE ("Прошили")) -> ()
            n300 = xnode "Read/Write Control"("FPGA VI Reference In"=w567, "W(T)/R(F)"="W(T)/R(F)", "Адрес"="Адрес", "Кол-во"="Кол-во") -> ("FPGA VI Reference Out"=w563:refnum<k20>)  [unwired: 1 in, 1 out]
          }
          frame #1 {
            n301 = Wait (ms)(milliseconds to wait=u32 1) -> ()  [unwired: 1 out]
          }
          frame #2 {
            n302 = xnode "Read/Write Control"("FPGA VI Reference In"=w570, "4-wire"=TRUE ("SPI")) -> ()  [unwired: 1 in, 2 out]
          }
          frame #3 {
            n303 = Wait (ms)(milliseconds to wait=u32 1) -> ()  [unwired: 1 out]
          }
          frame #4 {
            n304 = xnode "Read/Write Control"("FPGA VI Reference In"=w574, "4-wire"=FALSE ("SPI"), "Upd_RD"=TRUE) -> ()  [unwired: 1 in, 2 out]
          }
          frame #5 {
            n305 = Wait (ms)(milliseconds to wait=u32 1) -> ()  [unwired: 1 out]
          }
          frame #6 {
            n306 = xnode "Read/Write Control"("FPGA VI Reference In"=w577, "Upd_RD"=FALSE) -> ()  [unwired: 1 in, 2 out]
          }
          frame #7 {
            n307 = xnode "Invoke Method"("FPGA VI Reference In"=w581, "Number of Elements"=u32 0, "Timeout (ms)"=0) -> ("Elements Remaining"=w578:u32)  [unwired: 1 in, 3 out]
            "FIFO_READ" <- w578
          }
          frame #8 {
            n308 = xnode "Invoke Method"("FPGA VI Reference In"=w586, "Number of Elements"=w585, "Timeout (ms)"=0) -> ("Data"=→"READ":u8[])  [unwired: 1 in, 3 out]
            n309 = local read "Стоп"() -> (w587:bool)
            "Прошили" <- TRUE ("Прошили")
          }
        }
      }
    }
  }
  n310 = call <instrlib>:"niDCPower Close.vi"("instrument handle"=w1) -> ()  [unwired: 10 in, 1 out]
  n311 = call <instrlib>:"niDCPower Close.vi"("instrument handle"=w2) -> ()  [unwired: 10 in, 1 out]
  n312 = Close File(refnum=w17) -> ()  [unwired: 1 in, 2 out]
  n313 = flat-sequence {
    tunnel: w13 -> [_]
    tunnel: w9 -> [w589]
    tunnel: w7 -> [_]
    tunnel: w6 -> [_]
    tunnel: w5 -> [_]
    frame #0 {
      n314 = xnode "Read/Write Control"("FPGA VI Reference In"=w589, "Стоп"=TRUE) -> ("FPGA VI Reference Out"=w590:refnum<k20>)  [unwired: 1 in, 1 out]
      n315 = xnode "Close FPGA VI Reference"("FPGA VI Reference In"=w590) -> ()  [unwired: 1 in, 1 out]
    }
  }
